vi "test_headers_get_all.vi"() -> ()   [LabVIEW 2020, in "reqwest_tests.lvlib"]
uses:
  reqwest_tests.lvlib
  <vilib>/addons/_JKI Toolkits/Caraya/classes/Assert/Assert Equal Value_Variant.vi
  Headers/Headers.lvclass
  <vilib>/addons/_JKI Toolkits/Caraya/classes/Assert/Assert.lvclass
  <vilib>/addons/_JKI Toolkits/Caraya/classes/Test/Test.lvclass
panel:
  out "headers 2":cluster{"name":string, "value":string}[](array[cluster])
  out "headers":string
  out "success":bool
  in  "error in (no error)":errorcluster
  out "error out":errorcluster
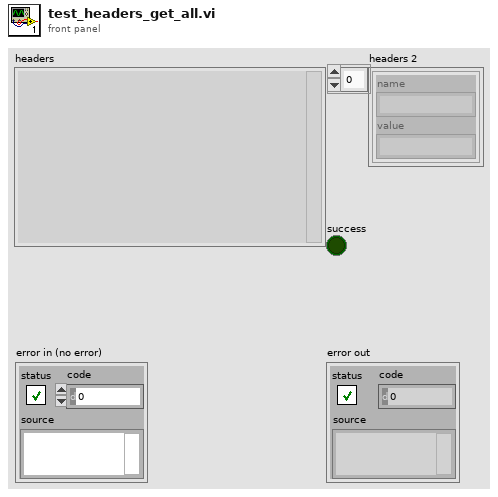
[diagram p1: front panel]
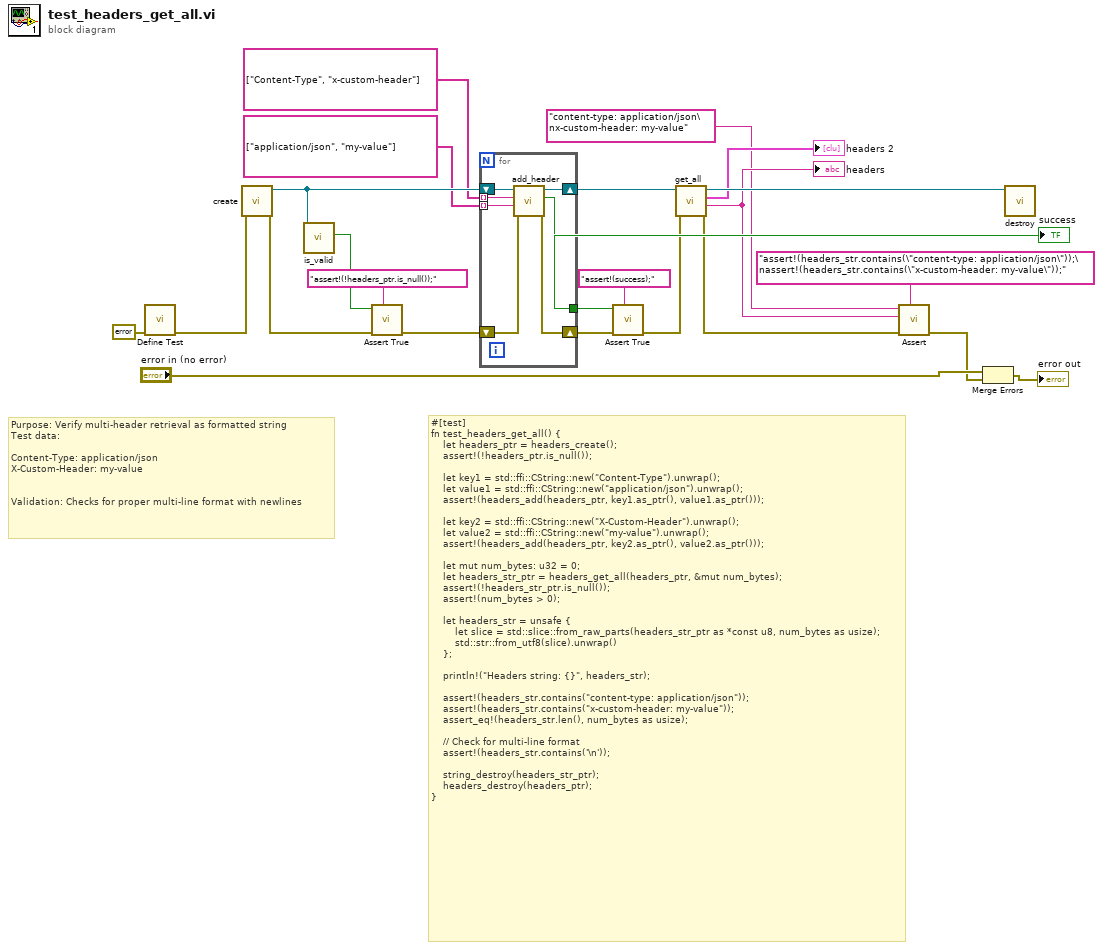
[diagram p0: block diagram]
diagram:
  # "Purpose: Verify multi-header retrieval as formatted string\nTest data:\n\nContent-Type: application/json\nX-Custom-Header: my-value\n\n\nValidation: Checks for proper multi-line format with newlines"
  # "#[test]\nfn test_headers_get_all() {\n    let headers_ptr = headers_create();\n    assert!(!headers_ptr.is_null());\n\n    let key1 = std::ffi::CString::new(\"Content-Type\").unwrap();\n    let value1 = std::ffi::CString::new(\"application/json\").unwrap();\n    assert!(headers_add(headers_ptr, key1.as_ptr(), value1.as_ptr()));\n\n    let key2 = std::ffi::CString::new(\"X-Custom-Header\").unwrap();\n    let value2 = std::ffi::CString::new(\"my-value\").unwrap();\n    assert!(headers_add(headers_ptr, key2.as_ptr(), value2.as_ptr()));\n\n    let mut num_bytes: u32 = 0;\n    let headers_str_ptr = headers_get_all(headers_ptr, &mut num_bytes);\n    assert!(!headers_str_ptr.is_null());\n    assert!(num_bytes > 0);\n\n    let headers_str = unsafe {\n        let slice = std::slice::from_raw_parts(headers_str_ptr as *const u8, num_bytes as usize);\n        std::str::from_utf8(slice).unwrap()\n    };\n\n    println!(\"Headers string: {}\", headers_str);\n\n    assert!(headers_str.contains(\"content-type: application/json\"));\n    assert!(headers_str.contains(\"x-custom-header: my-value\"));\n    assert_eq!(headers_str.len(), num_bytes as usize);\n\n    // Check for multi-line format\n    assert!(headers_str.contains('\\n'));\n\n    string_destroy(headers_str_ptr);\n    headers_destroy(headers_ptr);\n}"
  n1 = call <vilib>:"Define Test.vi"("error in (no error)"=errorcluster {"status"=FALSE, "code"=0, "source"=""}) -> ("error out"=w20:errorcluster)  [unwired: 9 in, 1 out]
  n2 = call "create.vi"("error in (no error)"=w20) -> ("error out"=w15:errorcluster, "Headers out"=w18:refnum<class "Headers.lvclass">)  [unwired: 9 in]
  n3 = call "is_valid.vi"("Headers in"=w18) -> ("valid-ref?"=w16:bool)  [unwired: 10 in]
  n4 = call <vilib>:"Assert True.vi"("Label"="assert!(!headers_ptr.is_null());", "error in (no error)"=w15, "True?"=w16) -> ("error out"=w14:errorcluster)  [unwired: 7 in, 1 out]
  n5 = for {
    tunnel: [w28] -> w7
    shift-right: [w27] -> w13
    shift-left: w18 -> [w30]
    shift-right: [w26] -> w8
    shift-left: w14 -> [w29]
    tunnel: string[] ["Content-Type", "x-custom-header"] ("key") -> [w25] mode=indexing
    tunnel: string[] ["application/json", "my-value"] ("key") -> [w24] mode=indexing
    n6 = call "add_header.vi"("error in (no error)"=w29, "value"=w24, "key"=w25, "Headers in"=w30) -> ("error out"=w26:errorcluster, "success"=w28:bool, "Headers out"=w27:refnum<class "Headers.lvclass">)  [unwired: 5 in]
  }
  "success" <- w7
  n7 = call <vilib>:"Assert True.vi"("Label"="assert!(success);", "error in (no error)"=w8, "True?"=w7) -> ("error out"=w6:errorcluster)  [unwired: 7 in, 1 out]
  n8 = call "get_all.vi"("error in (no error)"=w6, "Headers in"=w13) -> ("error out"=w5:errorcluster, 1:"headers"=w4:string, 2:"headers"=→"headers 2":cluster{"name":string, "value":string}[], "Headers in"=w12:refnum<class "Headers.lvclass">)  [unwired: 6 in]
  "headers" <- w4
  n9 = call-poly <vilib>:"Assert.vi"("Label"="assert!(headers_str.contains(\"content-type: application/json\"));\nassert!(headers_str.contains(\"x-custom-header: my-value\"));", "error in (no error)"=w5, "Y"=w4, "X"="content-type: application/json\nx-custom-header: my-value" ("key")) -> ("error out"=w2:errorcluster)  [unwired: 6 in, 1 out]
  n10 = Merge Errors("error in (no error)", w2) -> (→"error out":errorcluster)
  n11 = call "destroy.vi"("Headers in"=w12) -> ()  [unwired: 10 in, 1 out]
